vi "check result.vi"() -> ()   [LabVIEW 2015]
panel:
  in  "Graph 2":cluster{"X":dbl[], "y":dbl[]}[](graph)=[{"X"=array[902 elements], "y"=array[902 elements]}, {"X"=array[902 elements], "y"=array[902 elements]}, {"X"=[40.0, -6.0], "y"=[0.0, 0.0]}, {"X"=[0.0, 0.0], "y"=[80.0, -80.0]}]
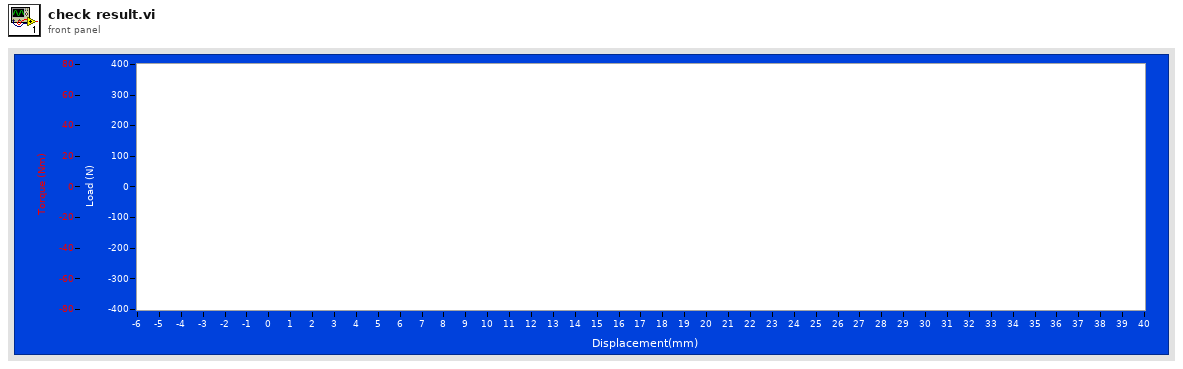
[diagram p1: front panel]
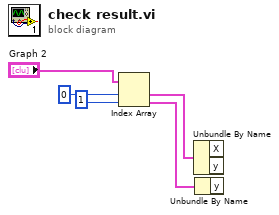
[diagram p0: block diagram]
diagram:
  n1 = Index Array(array="Graph 2", index #1=0 ("index"), index #2=1 ("index")) -> (element #1=w4:cluster{"X":dbl[], "y":dbl[]}, element #2=w1:cluster{"X":dbl[], "y":dbl[]})
  n2 = Unbundle By Name(w4) -> ()  [unwired: 2 out]
  n3 = Unbundle By Name(w1) -> ()  [unwired: 1 out]
